vi "DELETEGet SMO Address.vi"(8 "error in (no error)":errorcluster, 11 "Instrument.Template in":refnum<class "Instrument.Framework-Template.lvclass">) -> (0 "error out":errorcluster, 2 "SMO Address":string, 3 "Instrument.Template out":refnum<class "Instrument.Framework-Template.lvclass">)   [LabVIEW 2019]
uses:
  Instrument.Framework-Template.lvclass
  Framework/Instrument Types/SCPI/Instrument.SCPI.lvclass
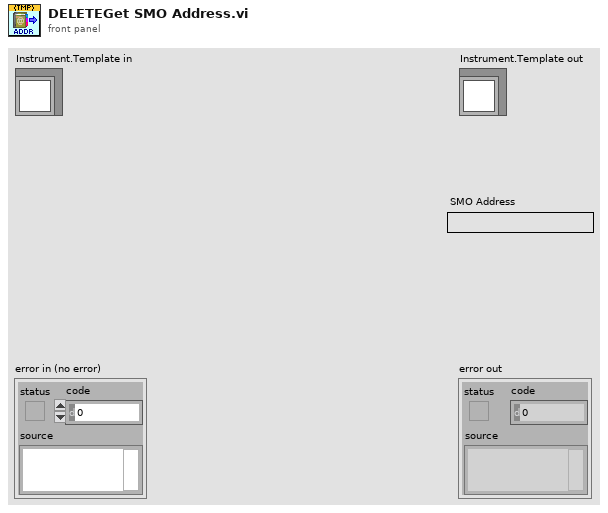
[diagram p1: front panel]
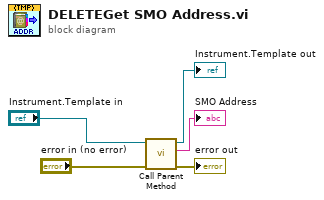
[diagram p0: block diagram]
diagram:
  n1 = call-parent "Call Parent Method"("error in (no error)"="error in (no error)", "Instrument in"="Instrument.Template in") -> ("error out"=→"error out":errorcluster, "SMO Address"=→"SMO Address":string, "Instrument out"=→"Instrument.Template out":refnum<class "Instrument.Framework-Template.lvclass">)  [unwired: 7 in]
